vi "1Main.vi"() -> ()   [LabVIEW 2014]
panel:
  in  "Stop Child":bool
  out "Boolean":bool
  out "i2":i32
  out "error out":errorcluster
  in  "launch":bool
  out "i":i32
  in  "Stop Button":bool
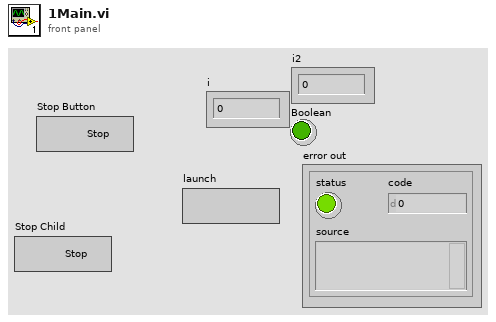
[diagram p1: front panel]
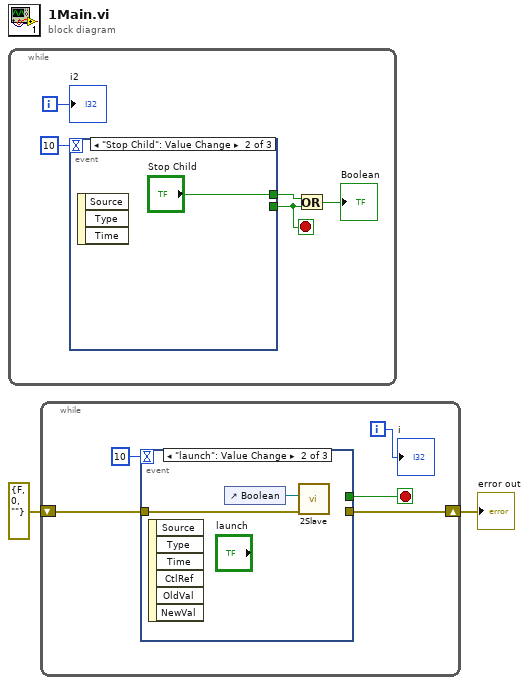
[diagram p0: block diagram]
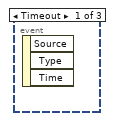
[diagram p2: hidden frame]
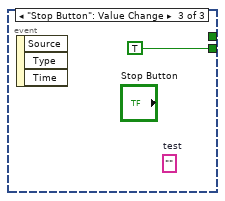
[diagram p3: hidden frame]
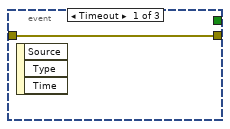
[diagram p4: hidden frame]
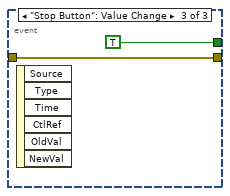
[diagram p5: hidden frame]
diagram:
  n1 = while {
    i -> [w7]
    stop <- w3 stop-if-true
    n2 = event shown="[1] \"Stop Child\": Value Change" {
      selector: _ -> [_ _ _]
      dyn-events: _ -> [_ _ _]
      timeout: 10 -> [_ _ _]
      tunnel: [_ _ TRUE] -> w3
      tunnel: [_ "Stop Child" _] -> w5
      event Timeout {
        n3 = event-data() -> ()  [unwired: 1 in, 3 out]
      }
      event "Stop Child": Value Change {
        n4 = event-data() -> ()  [unwired: 1 in, 3 out]
      }
      event "Stop Button": Value Change {
        (unwired) ""  # test
        n5 = event-data() -> ()  [unwired: 1 in, 3 out]
      }
    }
    n6 = Or(x=w5, y=w3) -> (x .or. y?=→"Boolean":bool)
    "i2" <- w7
  }
  n7 = while {
    shift-right: [w10] -> w2
    shift-left: errorcluster {"status"=FALSE, "code"=0, "source"=""} ("error out") -> [w11]
    i -> [w12]
    stop <- w13 stop-if-true
    n8 = event shown="[1] \"launch\": Value Change" {
      selector: _ -> [_ _ _]
      dyn-events: _ -> [_ _ _]
      timeout: 10 ("Numeric Control") -> [_ _ _]
      tunnel: [_ _ TRUE] -> w13
      tunnel: w11 -> [w15 w17 w18]
      tunnel: [w15 _ w18] -> w10
      event Timeout {
        n9 = event-data() -> ()  [unwired: 1 in, 3 out]
      }
      event "launch": Value Change {
        n10 = event-data() -> ()  [unwired: 1 in, 6 out]
        n11 = control-ref of="Boolean"() -> (w16:refnum<vi>)
        n12 = call "2Slave.vi"("error in (no error)"=w17, "Stop Ref"=w16) -> ()  [unwired: 9 in, 1 out]
      }
      event "Stop Button": Value Change {
        n13 = event-data() -> ()  [unwired: 1 in, 6 out]
      }
    }
    "i" <- w12
  }
  "error out" <- w2
